vi "Determine_region.vi"(9 "x2":dbl, 10 "x1":dbl) -> (2 "Region":dbl)   [LabVIEW 2016]
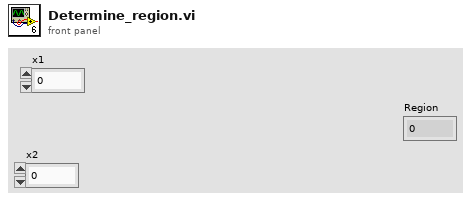
[diagram p1: front panel]
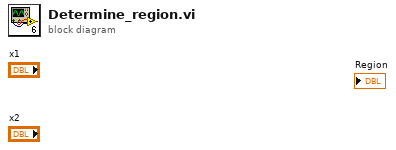
[diagram p0: block diagram]
diagram:
